vi "SparkMAXCommandPosition.vi"(0 "Device Reference (in)":T3, 5 "Output Mode":T1(ring), 7 "Control Mode":T2(ring), 9 "Position (counts) or Testing Power":dbl, 11 "Error (in)":errorcluster, 12 "Feed Forward Power [-1, 1]":dbl) -> ()   [LabVIEW 2023]
doc: "Wrapper for commanding the postion of a Talon FX motor controller. Supports PID, Motion Magic, and a safety interlock. Also supports the standard actuator testing interface and and the only sending new values on change."
uses:
  <vilib>/Rock Robotics/WPI/MotorControl/WPI_MotorControlDeviceRef.ctl
  <vilib>/Rock Robotics/WPI/MotorControl/WPI_MotorControlType.ctl
  <vilib>/Rock Robotics/SystemInterfaces/DIO/FPGA_DIOPWMChannel.ctl
  <vilib>/Rock Robotics/WPI/PWM/WPI_PWMDeadband.ctl
  <vilib>/Rock Robotics/SystemInterfaces/DIO/FPGA_DIOChannel.ctl
  <vilib>/Rock Robotics/WPI/ThirdParty/REV Robotics/REVLib/Typedef/Spark MAX Control Type.ctl
  <vilib>/Rock Robotics/WPI/ThirdParty/Phoenix-LabVIEW/Motor Controller/Controls/CTRE_Phoenix_MotorControl_ControlMode.ctl
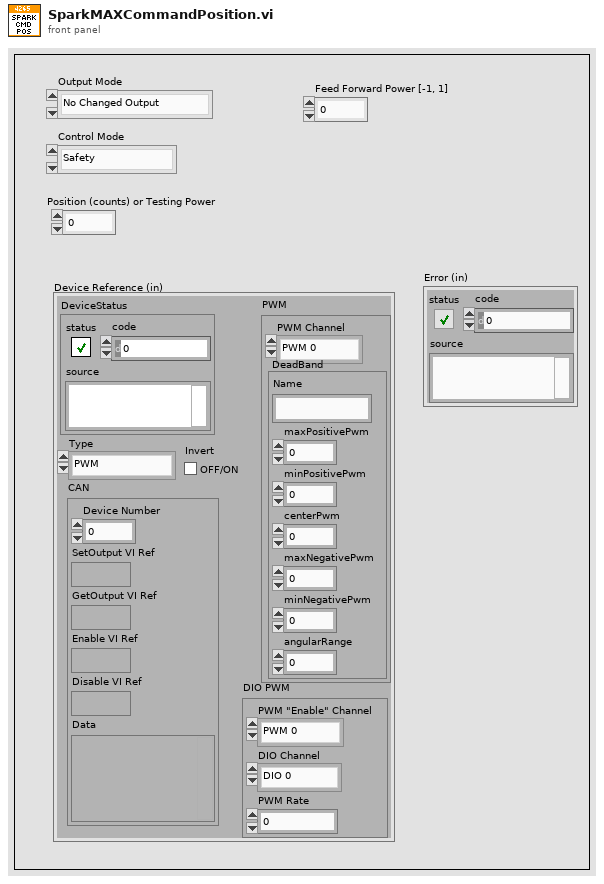
[diagram p1: front panel]
types:
  T1 = enum16{"No Changed Output", "New Normal Output", "New Testing Output"}
  T2 = enum16{"Safety", "Travelling", "Positioning", "Holding"}
  T3 = typedef "WPI_MotorControlDeviceRef.ctl" = cluster{"DeviceStatus":errorcluster, "Type":T4, "PWM":cluster{"PWM Channel":T5, "DeadBand":T6}, "CAN":cluster{"Device Number":u8, "SetOutput VI Ref":variant, "GetOutput VI Ref":variant, "Enable VI Ref":variant, "Disable VI Ref":variant, "Data":variant}, "Invert":bool, "DIO PWM":cluster{"PWM \"Enable\" Channel":T5, "DIOChannel":T7, "PWM Rate":dbl}}
  T4 = typedef "WPI_MotorControlType.ctl" = enum16{"PWM", "CAN", "DIO PWM"}
  T5 = typedef "FPGA_DIOPWMChannel.ctl" = enum8{"PWM 0", "PWM 1", "PWM 2", "PWM 3", "PWM 4", "PWM 5", "PWM 6", "PWM 7", "PWM 8", "PWM 9", "PWM MXP 0", "PWM MXP 1", "PWM MXP 2", "PWM MXP 3", "PWM MXP 4", "PWM MXP 5", "PWM MXP 6", "PWM MXP 7", "PWM MXP 8", "PWM MXP 9", "Invalid"}
  T6 = typedef "WPI_PWMDeadband.ctl" = cluster{"Name":string, "maxPositivePwm":i32, "minPositivePwm":i32, "centerPwm":i32, "maxNegativePwm":i32, "minNegativePwm":i32, "angularRange":u16}
  T7 = typedef "FPGA_DIOChannel.ctl" = enum8{"DIO 0", "DIO 1", "DIO 2", "DIO 3", "DIO 4", "DIO 5", "DIO 6", "DIO 7", "DIO 8", "DIO 9", "DIO MXP 0", "DIO MXP 1", "DIO MXP 2", "DIO MXP 3", "DIO MXP 4", "DIO MXP 5", "DIO MXP 6", "DIO MXP 7", "DIO MXP 8", "DIO MXP 9", "DIO MXP 10", "DIO MXP 11", "DIO MXP 12", "DIO MXP 13", "DIO MXP 14", "DIO MXP 15", "SPI Port CS1", "SPI Port CS2", "SPI Port CS3", "SPI Port MISO", "SPI Port MOSI", "Invalid"}
  T8 = typedef "Spark MAX Control Type.ctl" = enum16{"Percent VBus", "Voltage", "Velocity", "Position", "Smart Motion", "Current", "Smart Velocity"}
  T9 = typedef "CTRE_Phoenix_MotorControl_ControlMode.ctl" = u16
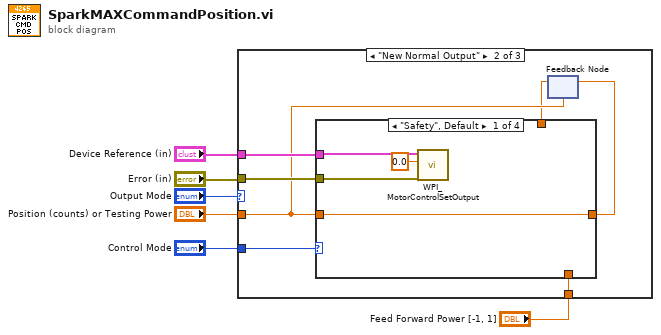
[diagram p0: block diagram]
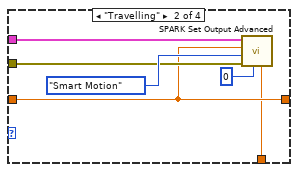
[diagram p3: hidden frame]
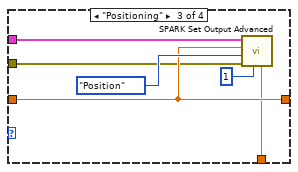
[diagram p4: hidden frame]
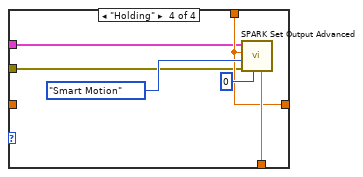
[diagram p5: hidden frame]
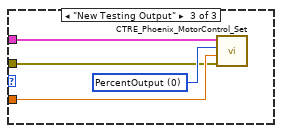
[diagram p6: hidden frame]
diagram:
  n1 = case shown="\"New Normal Output\"" "Output Mode" {
    tunnel: "Position (counts) or Testing Power" -> [_ w9 w38]
    tunnel: "Device Reference (in)" -> [_ w12 w39]
    tunnel: "Feed Forward Power [-1, 1]" -> [_ w13 _]
    tunnel: "Control Mode" -> [_ w11 _]
    tunnel: "Error (in)" -> [_ w10 w36]
    frame "No Changed Output", Default {
    }
    frame "New Normal Output" {
      n2 = feedback #1(w9) -> (w7:dbl)
      n3 = case shown="\"Safety\", Default" w11 {
        tunnel: w12 -> [w16 w21 w25 w31]
        tunnel: w9 -> [w17 w19 w27 _]
        tunnel: w13 -> [_ w18 w26 w33]
        tunnel: w10 -> [w15 w20 w24 w30]
        tunnel: [w17 w19 w27 w32] -> w8
        tunnel: w7 -> [_ _ _ w32]
        frame "Safety", Default {
          n4 = call <vilib>:"WPI_MotorControlSetOutput.vi"("error in (no error)"=w15, "Output"=0.0, "MotorControlDevRef"=w16) -> ()  [unwired: 6 in, 3 out]
        }
        frame "Travelling" {
          n5 = call <vilib>:"SPARK Set Output Advanced.vi"("Arbitrary Feed Forward (0)"=w18, "PIDF Slot (0)"=0, "error in (no error)"=w20, "Control Mode"=Spark_MAX_Control_Type."Smart Motion", "Setpoint"=w19, "MotorControlDevRef"=w21) -> ()  [unwired: 4 in, 2 out]
        }
        frame "Positioning" {
          n6 = call <vilib>:"SPARK Set Output Advanced.vi"("Arbitrary Feed Forward (0)"=w26, "PIDF Slot (0)"=1, "error in (no error)"=w24, "Control Mode"=Spark_MAX_Control_Type."Position", "Setpoint"=w27, "MotorControlDevRef"=w25) -> ()  [unwired: 4 in, 2 out]
        }
        frame "Holding" {
          n7 = call <vilib>:"SPARK Set Output Advanced.vi"("Arbitrary Feed Forward (0)"=w33, "PIDF Slot (0)"=0, "error in (no error)"=w30, "Control Mode"=Spark_MAX_Control_Type."Smart Motion", "Setpoint"=w32, "MotorControlDevRef"=w31) -> ()  [unwired: 4 in, 2 out]
        }
      }
      n8 = feedback-in #1(w8) -> ()
    }
    frame "New Testing Output" {
      w37 = T9 0 items=["PercentOutput"=0, "Position"=1, "Velocity"=2, "Current"=3, "Follower"=5, "MotionProfile"=6, "MotionMagic"=7, "MotionProfileArc"=10, "Disabled"=15] ("Control Mode")
      n9 = call <vilib>:"CTRE_Phoenix_MotorControl_Set.vi"("error in (no error)"=w36, "Output"=w38, "Control Mode"=w37, "PhoenixMotorControlDevRef"=w39) -> ()  [unwired: 6 in, 2 out]
    }
  }
